vi "Demo String and Numeric.vi"(8 "error in (no error)":errorcluster) -> (0 "error out":errorcluster)   [LabVIEW 2011]
uses:
  VIremote.llb/VIremoteEvent.ctl
  VIremote.llb/VIremoteFunction.ctl
panel:
  in  "Color Box":u32(colorbox)=33023
  in  "VIremoteEvent":T1=enum."Connection Closed"
  in  "Single Line String":string="Tap here" caption="Single Line"
  in  "Numeric":dbl format="%#.1f"
  in  "Multi Line String":string="Tap here"
  # "Tap a string control to bring up the keyboard. If a control has \"Limit to Single Line\" set then the Return key will be replaced by a Done key which will dismiss the keyboard. When a control loses key focus the keyboard will allways dismiss."
  # "Tap a numeric control to bring up the numeric keyboard.\nThis control has been customized with bigger up/down buttons so they are easier to hit.\nColor Box will display popup with thre sliders for red green blue."
  # "Auto scroll enabled: If a control with key focus is hidden by the keyboard it will be scrolled into view. This is true for the numeric control above."
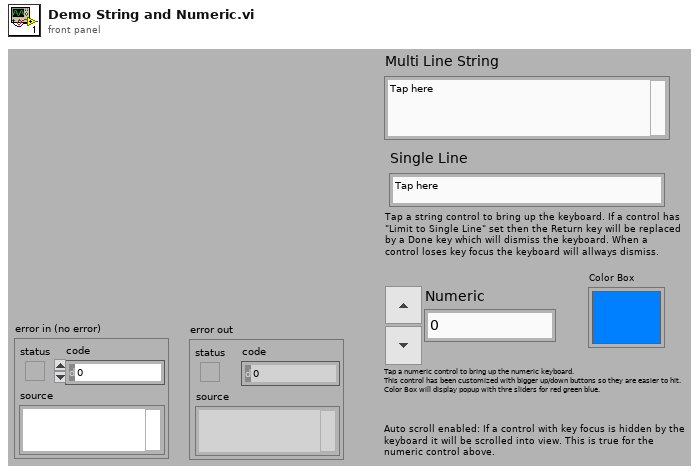
[diagram p1: front panel]
types:
  T1 = typedef "VIremoteEvent.ctl" = enum16{"No Event", "Connection Closed", "Navigate Back", "Enter Background", "Enter Foreground", "Portrait", "Portrait Upside Down", "Landscape Left", "Landscape Right"}
  T2 = typedef "VIremoteFunction.ctl" = enum16{"Do nothing", "Stop controller", "Close this connection", "Show info panel", "Set VI to control", "Set Accelerometer freq (Hz)", "Show Alert message", "Start Sound Input", "Stop Sound Input", "Set Volume (0-100)", "Set sound output Speaker", "Set sound output Receiver", "Play Sound", "Repeat Sound", "Stop Sound", "Pause Sound", "Resume Sound", "Set panel width of caller (320 or 480)", "Set Panel Size to Portrait", "Set Panel Size to Landscape", "Set Panel Size as Current Orientation", "Allow all UI Orientations", "Send user notification", "Disable Scrolling", "Normal Scrolling", "Page Scrolling", "Set Scroll Offset", "Page Indicator Position"}
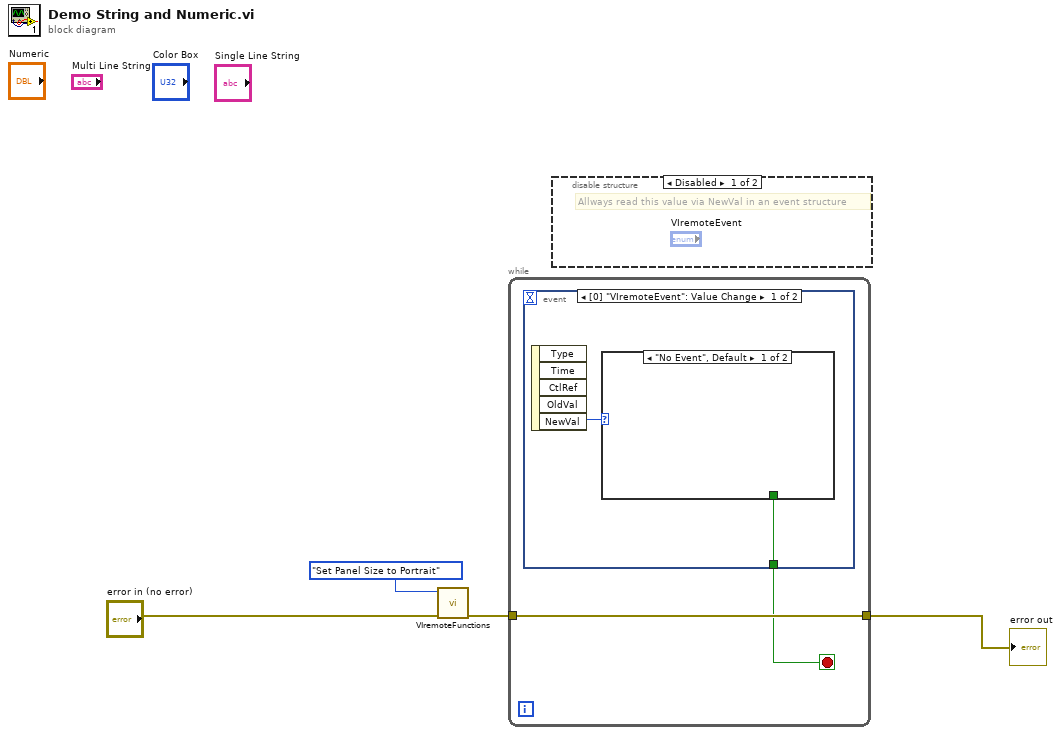
[diagram p0: block diagram]
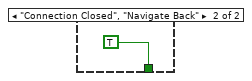
[diagram p3: hidden frame]
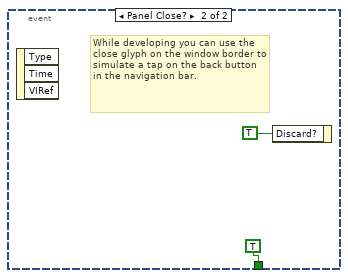
[diagram p4: hidden frame]
diagram:
  n1 = call "VIremoteFunctions.vi"("error in (no error)"="error in (no error)", "Function"=VIremoteFunction."Set Panel Size to Portrait") -> ("error out"=w3:errorcluster)  [unwired: 4 in, 5 out]
  n2 = while {
    tunnel: [w6] -> w1
    tunnel: w3 -> [w6]
    stop <- w5 stop-if-true
    n3 = event shown="[0] \"VIremoteEvent\": Value Change" {
      selector: _ -> [_ _]
      dyn-events: _ -> [_ _]
      timeout: _ -> [_ _]
      tunnel: [w7 TRUE] -> w5
      event Value Change {
        n4 = event-data() -> ("NewVal"=w8:T1)  [unwired: 5 out]
        n5 = case shown="\"No Event\", Default" w8 {
          tunnel: [_ TRUE] -> w7
          frame "No Event", Default {
          }
          frame "Connection Closed", "Navigate Back" {
          }
        }
      }
      event Panel Close? {
        # "While developing you can use the close glyph on the window border to simulate a tap on the back button in the navigation bar."
        n6 = event-data() -> ()  [unwired: 4 out]
        n7 = event-data("Discard?"=TRUE) -> ()  [unwired: 1 in, 1 out]
      }
    }
  }
  "error out" <- w1
  n8 = disable-structure shown="Disabled" {
    frame Disabled {
      # "Allways read this value via NewVal in an event structure"
    }
    frame Enabled {
    }
  }
